vi "Evaluate.vi"(8 "error in (no error)":errorcluster, 11 "Expectation in":refnum<class "Expectation.lvclass">) -> (0 "error out":errorcluster, 1 "Message":string, 2 "Passed?":bool)   [LabVIEW 2020, in "Expectation.lvclass"]
uses:
  Expectation.lvclass
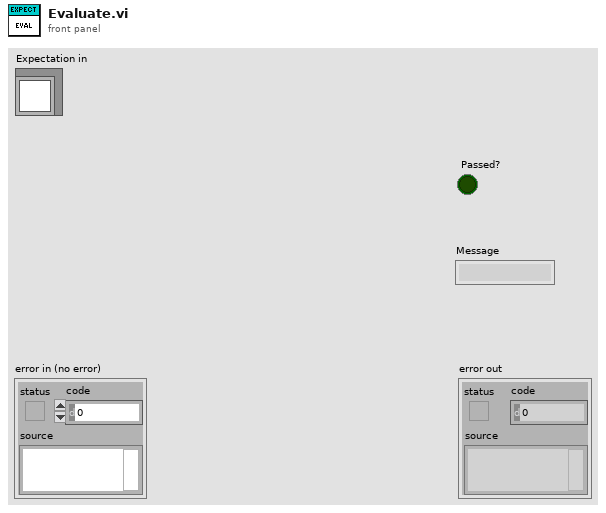
[diagram p1: front panel]
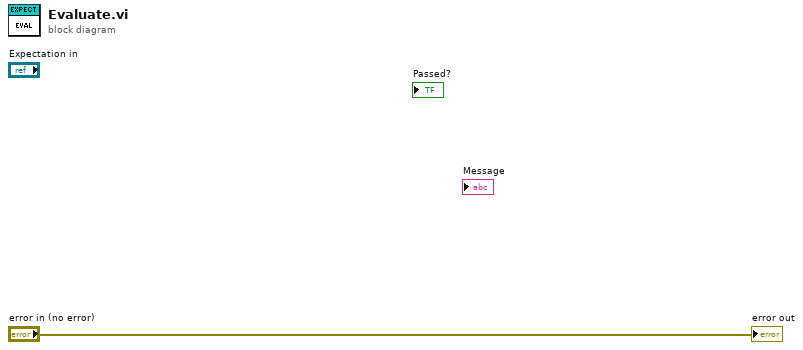
[diagram p0: block diagram]
diagram:
  "error out" <- "error in (no error)"
